vi "util_is_in_array.vi"(2 "Array":dbl[](array[numeric]), 3 "Numeric":dbl format="%#_13g") -> (0 "Position":i32, 1 "Contains element?":bool)   [LabVIEW 2020]
doc: "Check if array contains a certain value and return its position."
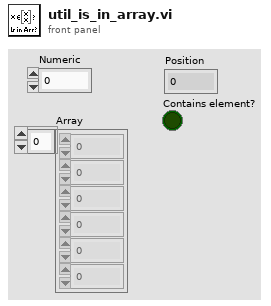
[diagram p1: front panel]
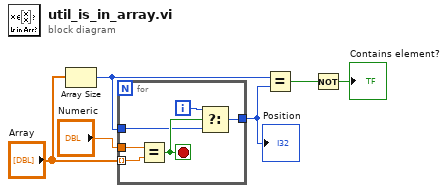
[diagram p0: block diagram]
diagram:
  n1 = Array Size(array="Array") -> (size(s)=w4:i32)
  n2 = for {
    tunnel: "Array" -> [w11] mode=indexing
    tunnel: "Numeric" -> [w12]
    tunnel: w4 -> [w7]
    tunnel: [w9] -> w3
    i -> [w10]
    stop <- w8 stop-if-true
    n3 = Equal?(x=w12, y=w11) -> (x = y?=w8:bool)
    n4 = Select(t=w10, s=w8, f=w7) -> (s? t:f=w9:i32)
  }
  "Position" <- w3
  n5 = Equal?(x=w4, y=w3) -> (x = y?=w2:bool)
  n6 = Not(x=w2) -> (.not. x?=→"Contains element?":bool)
